vi "FGV ARN Daten.vi"(0 "ARN Konfig Daten":T1={"Bearbeiter:"="", "Analysator"="FT-IR", "Komponente:"=0, "Gasflaschen Nr.:"="", "Accuracy"=0.0, "Sollwert"=0.0, "Modus"=0, "Pfad:"=path "D:/IAG_Data/Log", "Textname:"="", "CG Aufschaltzeit:"=120.0, "Einheit"="", "N2 Aufschaltzeit:"=120.0, "Gasflasche"=0, "Konfig Gasflasche"=FALSE} {"Gasflasche" items=["----"=10000, "IAG NH3 3000"=0, "IAG NH3 200"=1, "IAG NH3 2000"=2, "IAG MG"=3, "IAG O2"=4]; "Komponente:" items=["NO (350,3000) LP 191C", "NO2 (150) LP 191C (1of2)", "NO2 (2000) LP 191C (2of2)", "N2O (300) LP 191C (1of2)", "NH3 (300) LP 191C (1of2)", "NH3 (900,3000) LP 191C (2of2)", "HNCO (400) 191C", "H2O% (30) LP 191C", "Formaldehyde (70,500) LP 191C", "CO2 low% (4) LP 191C (2of2)", "CO2% (20) LP 191C (1of2)", "CO (700) LP 191C (1of3)", "CO% (1) LP 191C (2of3)", "Propylene (1000) LP 191C", "Aromatic HC C7 (500) LP 191C", "Ethylene (1000) LP 191C", "CH4 (250) LP 191C (1of2)", "CH4 (5000) LP 191C (2of2)", "Ethane (1000) LP 191C", "Acetylene (1000) LP 191C", "HNO2 (20) 191C", "MeOH (1000) 191C", "CO% (10) LP 191C (3of3)", "Formic Acid (100) 191C", "SO2 (500) LP 191C", "Acetaldehyde (1000) LP 191C", "COS (100) LP 191C", "1,3 butadiene (100) LP 191C", "Oil as Octane (200) LP 191C", "N2O (1000) LP 191C (2of2)", "Propane (200) LP 191C", "NO2 autorange (2000)", "CO autorange (100000)", "CH4 autorange (5000)", "NH3 autorange (3000)", "Temp. Gascell", "Pressure Gascell", "sBeam@2500"]; "Modus" items=["CG zu PNS", "CG zu Entnahmestelle"]; "N2 Aufschaltzeit:" min=10.0; "CG Aufschaltzeit:" min=10.0}, 1 "N2":bool, 5 "Rohdaten":sgl[](array[numeric]), 7 "Zeitstempel":string, 9 "SNR Ergebnis":sgl[](array[numeric]), 11 "error in (no error)":errorcluster caption="Fehler (Eingang, kein Fehler)", 12 "Aktion":T6) -> (4 "ARN Konfig Daten":T1={"Bearbeiter:"="", "Analysator"="FT-IR", "Komponente:"=0, "Gasflaschen Nr.:"="", "Accuracy"=0.0, "Sollwert"=0.0, "Modus"=0, "Pfad:"=path "D:/IAG_Data/Log", "Textname:"="", "CG Aufschaltzeit:"=120.0, "Einheit"="", "N2 Aufschaltzeit:"=120.0, "Gasflasche"=0, "Konfig Gasflasche"=FALSE} {"Gasflasche" items=["----"=10000, "IAG NH3 3000"=0, "IAG NH3 200"=1, "IAG NH3 2000"=2, "IAG MG"=3, "IAG O2"=4]; "Komponente:" items=["NO (350,3000) LP 191C", "NO2 (150) LP 191C (1of2)", "NO2 (2000) LP 191C (2of2)", "N2O (300) LP 191C (1of2)", "NH3 (300) LP 191C (1of2)", "NH3 (900,3000) LP 191C (2of2)", "HNCO (400) 191C", "H2O% (30) LP 191C", "Formaldehyde (70,500) LP 191C", "CO2 low% (4) LP 191C (2of2)", "CO2% (20) LP 191C (1of2)", "CO (700) LP 191C (1of3)", "CO% (1) LP 191C (2of3)", "Propylene (1000) LP 191C", "Aromatic HC C7 (500) LP 191C", "Ethylene (1000) LP 191C", "CH4 (250) LP 191C (1of2)", "CH4 (5000) LP 191C (2of2)", "Ethane (1000) LP 191C", "Acetylene (1000) LP 191C", "HNO2 (20) 191C", "MeOH (1000) 191C", "CO% (10) LP 191C (3of3)", "Formic Acid (100) 191C", "SO2 (500) LP 191C", "Acetaldehyde (1000) LP 191C", "COS (100) LP 191C", "1,3 butadiene (100) LP 191C", "Oil as Octane (200) LP 191C", "N2O (1000) LP 191C (2of2)", "Propane (200) LP 191C", "NO2 autorange (2000)", "CO autorange (100000)", "CH4 autorange (5000)", "NH3 autorange (3000)", "Temp. Gascell", "Pressure Gascell", "sBeam@2500"]; "Modus" items=["CG zu PNS", "CG zu Entnahmestelle"]; "N2 Aufschaltzeit:" min=10.0; "CG Aufschaltzeit:" min=10.0}, 6 "Rohdaten":sgl[][](array[numeric]), 8 "Zeitstempel":string, 10 "SNR Ergebnis":sgl[](array[numeric]), 14 "Rohdaten N2":sgl[][](array[numeric]), 15 "error out":errorcluster caption="Fehler (Ausgang)")   [LabVIEW 2020, in "EPA 1065.lvlib" / "ARN Test 1065-305.lvlib"]
uses:
  ARN Test 1065-305.lvlib
  Aktion FGV ARN Daten.ctl
  Allgemeine Einstellungen.ctl
  Seiten/System Einstellungen V2/Analysatoren.ctl
  T90 1065-308/Modus.ctl
  Seiten/System Einstellungen V2/Gasflasche Auswahl.ctl
  Seiten/System Einstellungen V2/Konfig Gasflasche.ctl
  Allgemein/allgemeine Sub-VIs.lvlib
  T90 1065-308/T90 Test 1065-308.lvlib
  Seiten/System Einstellungen V2/System Einstellungen V2.lvlib
panel:
  # "%"
  # "sec."
  # "sec."
  # "%"
  # "sec."
  # "sec."
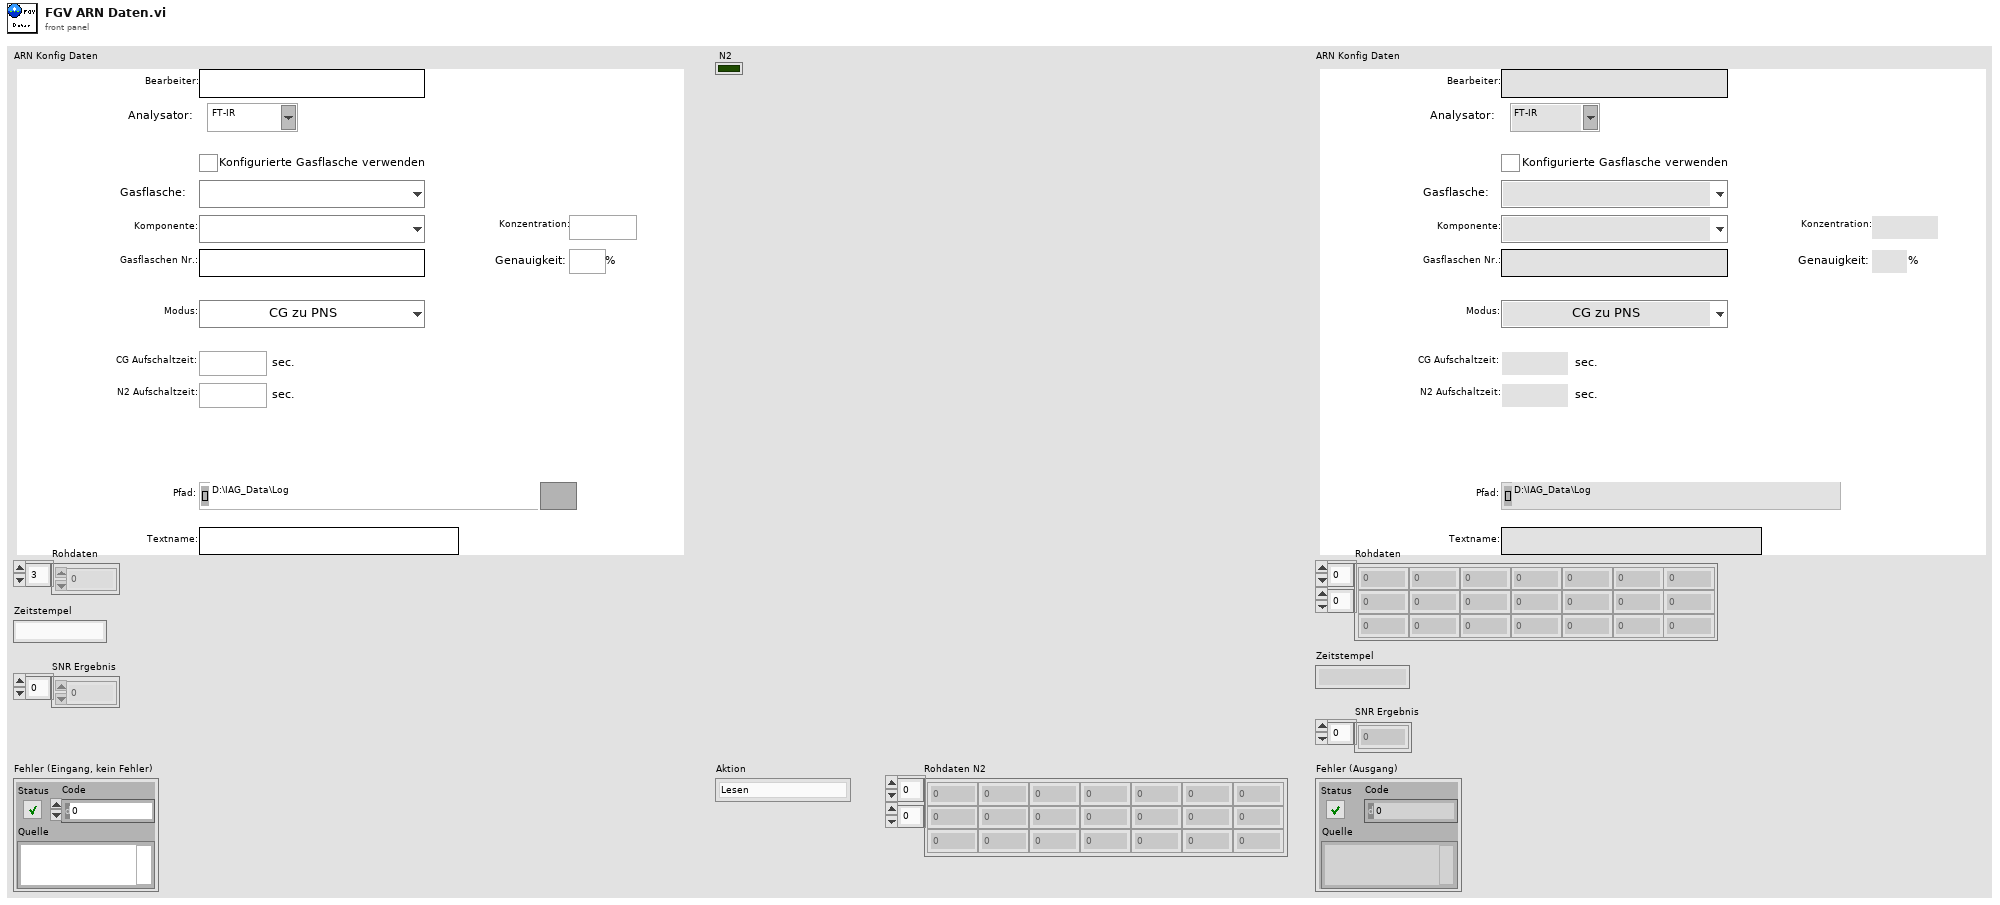
[diagram p1: front panel]
types:
  T1 = typedef "EPA 1065.lvlib/ARN Test 1065-305.lvlib/Allgemeine Einstellungen.ctl" = cluster{"Bearbeiter:":string, "Analysator":T2, "Komponente:":u16, "Gasflaschen Nr.:":string, "Accuracy":dbl, "Sollwert":dbl, "Modus":T3, "Pfad:":path, "Textname:":string, "CG Aufschaltzeit:":dbl, "Einheit":string, "N2 Aufschaltzeit:":dbl, "Gasflasche":T4, "Konfig Gasflasche":T5}
  T2 = typedef "System Einstellungen V2.lvlib/Analysatoren.ctl" = string
  T3 = typedef "EPA 1065.lvlib/T90 Test 1065-308.lvlib/Modus.ctl" = u16
  T4 = typedef "System Einstellungen V2.lvlib/Gasflasche Auswahl.ctl" = u16
  T5 = typedef "System Einstellungen V2.lvlib/Konfig Gasflasche.ctl" = bool
  T6 = typedef "EPA 1065.lvlib/ARN Test 1065-305.lvlib/Aktion FGV ARN Daten.ctl" = enum16{"Lesen", "laden", "speichern", "ARN Daten", "Rohdaten", "Rohdaten löschen", "Zeitstempel", "SNR Ergebnis"}
  T7 = enum16{"open", "replace", "create", "open or create", "replace or create", "replace or create with confirmation"}
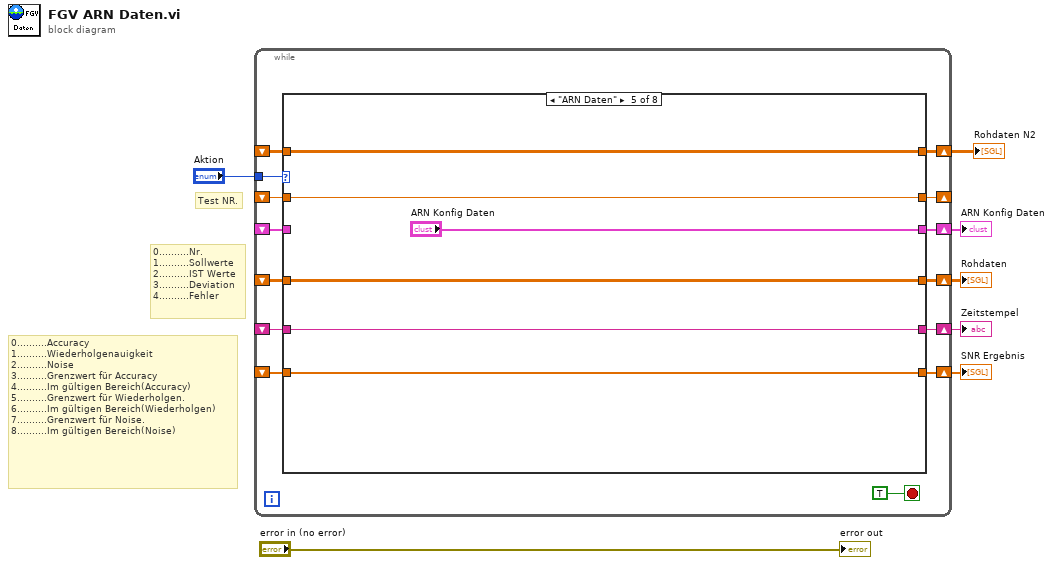
[diagram p0: block diagram]
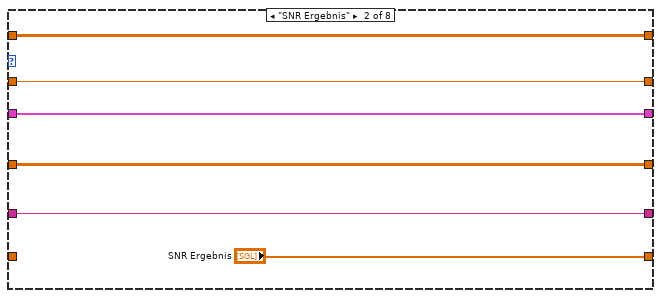
[diagram p3: hidden frame]
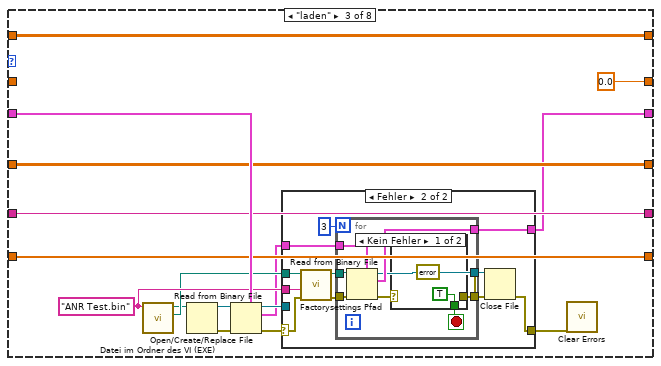
[diagram p4: hidden frame]
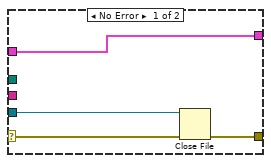
[diagram p5: hidden frame]
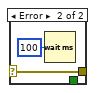
[diagram p6: hidden frame]
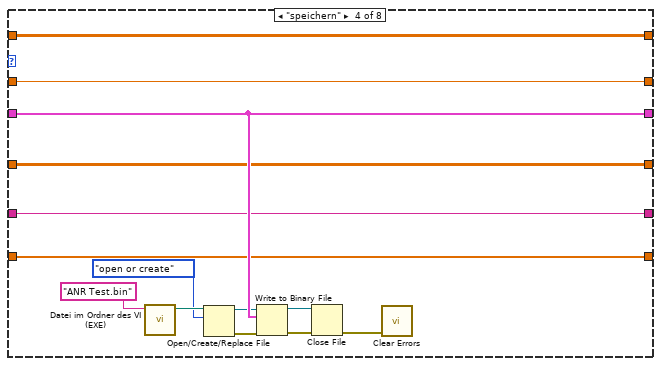
[diagram p7: hidden frame]
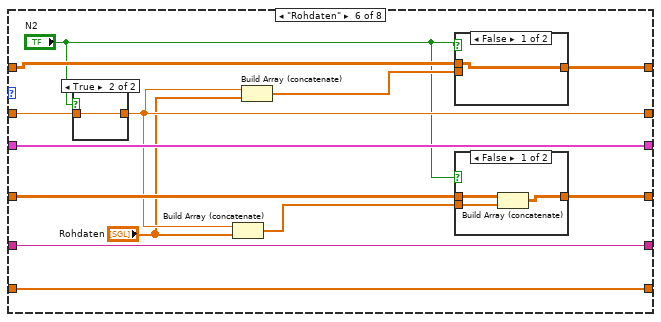
[diagram p8: hidden frame]
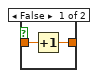
[diagram p10: hidden frame]
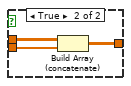
[diagram p11: hidden frame]
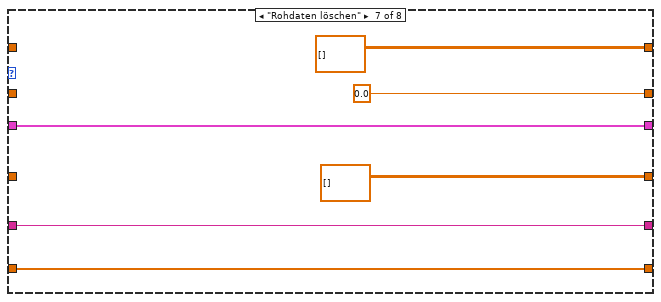
[diagram p12: hidden frame]
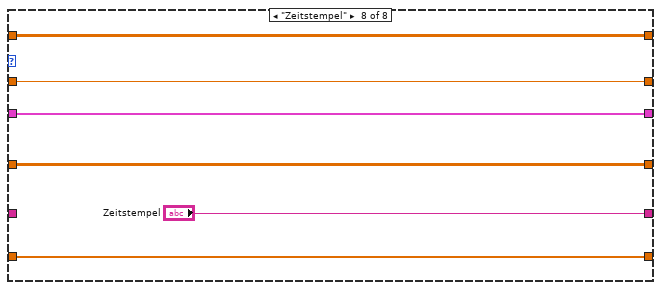
[diagram p13: hidden frame]
diagram:
  # "Test NR."
  # "0..........Accuracy\n1..........Wiederholgenauigkeit\n2..........Noise\n3..........Grenzwert für Accuracy\n4..........Im gültigen Bereich(Accuracy)\n5..........Grenzwert für Wiederholgen.\n6..........Im gültigen Bereich(Wiederholgen)\n7..........Grenzwert für Noise.\n8..........Im gültigen Bereich(Noise)"
  # "0..........Nr.\n1..........Sollwerte\n2..........IST Werte\n3..........Deviation\n4..........Fehler"
  n1 = while {
    tunnel: "Aktion" -> [w20]
    shift-right: [w19] -> w6
    shift-left: _ -> [w18]
    shift-right: [w17] -> w5
    shift-left: _ -> [w16]
    shift-right: [w15] -> w4
    shift-left: _ -> [w14]
    shift-right: [w13] -> w3
    shift-left: _ -> [w12]
    shift-right: [w11] -> _
    shift-left: _ -> [w10]
    shift-right: [w9] -> w1
    shift-left: _ -> [w8]
    stop <- TRUE stop-if-true
    n2 = case shown="\"ARN Daten\"" w20 {
      tunnel: [w27 w33 w38 w89 "ARN Konfig Daten" w109 w126 w132] -> w19
      tunnel: w18 -> [w27 w33 w49 w89 _ w109 w126 w132]
      tunnel: [w26 w32 w48 w88 w95 w103 sgl[][] [] ("Rohdaten") w131] -> w17
      tunnel: w16 -> [w26 w32 w48 w88 w95 w108 _ w131]
      tunnel: [w25 w31 w47 w87 w94 w107 w124 "Zeitstempel"] -> w15
      tunnel: w14 -> [w25 w31 w47 w87 w94 w107 w124 _]
      tunnel: [w24 "SNR Ergebnis" w46 w86 w93 w106 w123 w129] -> w13
      tunnel: w12 -> [w24 _ w46 w86 w93 w106 w123 w129]
      tunnel: [w23 w29 sgl 0.0 w85 w92 w102 sgl 0.0 w128] -> w11
      tunnel: w10 -> [w23 w29 _ w85 w92 w104 _ w128]
      tunnel: [w22 w28 w37 w84 w91 w99 sgl[][] [] w127] -> w9
      tunnel: w8 -> [w22 w28 w37 w84 w91 w98 _ w127]
      frame "Lesen", Default {
      }
      frame "SNR Ergebnis" {
      }
      frame "laden" {
        w42 = "ANR Test.bin" ("Dateiname")
        n3 = call "Datei im Ordner des VI (EXE).vi"("Dateiname"=w42) -> ("Ordner des Haupt-VIs"=w41:path, "Dateipfad im Ordner des Haupt-VIs"=w36:path)  [unwired: 8 in, 1 out]
        n4 = Open/Create/Replace File(file path (use dialog)=w36) -> (refnum out=w34:refnum<file>, error out=w35:errorcluster)  [unwired: 5 in, 1 out]
        n5 = Read from Binary File(5:w49, 8:w35, 11:w34) -> (0:w44:errorcluster, 2:w39:T1, 3:w40:refnum<file>)  [unwired: 3 in, 1 out]
        n6 = case shown="Fehler" w44 {
          selector: w44 -> [w52 w56]
          tunnel: w41 -> [_ w57]
          tunnel: w39 -> [w53 w55]
          tunnel: [w53 w63] -> w38
          tunnel: [w50 w61] -> w43
          tunnel: w40 -> [w51 _]
          tunnel: w42 -> [_ w54]
          frame No Error {
            n7 = Close File(refnum=w51, error in=w52) -> (error out=w50:errorcluster)  [unwired: 1 out]
          }
          frame Error {
            n8 = call "Factorysettings Pfad.vi"("error in (no error)"=w56, "Dateiname"=w54, "Ordner des Haupt-VIs"=w57) -> ("error out"=w58:errorcluster, "Pfad Factorysettings"=w59:path)  [unwired: 7 in]
            n9 = for {
              N: 3 -> [_]
              tunnel: w58 -> [w70]
              tunnel: w59 -> [w69]
              tunnel: [w68] -> w63
              tunnel: [w67] -> w62
              tunnel: [w66] -> w60
              tunnel: w55 -> [w65]
              stop <- w71 stop-if-true
              n10 = Read from Binary File(5:w65, 8:w70, 11:w69) -> (0:w72:errorcluster, 2:w68:T1, 3:w66:refnum<file>)  [unwired: 3 in, 1 out]
              n11 = case shown="Kein Fehler" w72 {
                selector: w72 -> [_ w75]
                tunnel: [TRUE _] -> w71
                tunnel: [errorcluster {"status"=FALSE, "code"=0, "source"=""} ("error IO") w75] -> w67
                frame No Error {
                }
                frame Error {
                  n12 = Wait (ms)(milliseconds to wait=u32 100 ("Zu wartende ms")) -> ()  [unwired: 1 out]
                }
              }
            }
            n13 = Close File(refnum=w60, error in=w62) -> (error out=w61:errorcluster)  [unwired: 1 out]
          }
        }
        n14 = call <vilib>:"Clear Errors.vi"("error in (no error)"=w43) -> ()  [unwired: 5 in, 2 out]
      }
      frame "speichern" {
        n15 = call "Datei im Ordner des VI (EXE).vi"("Dateiname"="ANR Test.bin") -> ("Dateipfad im Ordner des Haupt-VIs"=w82:path)  [unwired: 8 in, 2 out]
        n16 = Open/Create/Replace File(file path (use dialog)=w82, operation (0:open)=T7."open or create" ("Operation (0:Öffnen)")) -> (refnum out=w81:refnum<file>, error out=w83:errorcluster)  [unwired: 4 in, 1 out]
        n17 = Write to Binary File(file (use dialog)=w81, data=w89, error in=w83) -> (refnum out=w80:refnum<file>, error out=w79:errorcluster)  [unwired: 3 in, 1 out]
        n18 = Close File(refnum=w80, error in=w79) -> (error out=w78:errorcluster)  [unwired: 1 out]
        n19 = call <vilib>:"Clear Errors.vi"("error in (no error)"=w78) -> ()  [unwired: 5 in, 2 out]
      }
      frame "ARN Daten" {
      }
      frame "Rohdaten" {
        n20 = case shown="True" "N2" {
          tunnel: w104 -> [w115 w116]
          tunnel: [w114 w116] -> w102
          frame False {
            n21 = Increment(x=w115) -> (x+1=w114:sgl)
          }
          frame True {
          }
        }
        n22 = Build Array (concatenate)(w102, "Rohdaten") -> (w105:sgl[])
        n23 = Build Array (concatenate)(w102, "Rohdaten") -> (w100:sgl[])
        n24 = case shown="False" "N2" {
          tunnel: w100 -> [_ w120]
          tunnel: [w117 w119] -> w99
          tunnel: w98 -> [w117 w118]
          frame False {
          }
          frame True {
            n25 = Build Array (concatenate)(w118, w120) -> (w119:sgl[][])
          }
        }
        n26 = case shown="False" "N2" {
          tunnel: w108 -> [w112 w113]
          tunnel: w105 -> [w111 _]
          tunnel: [w110 w113] -> w103
          frame False {
            n27 = Build Array (concatenate)(w112, w111) -> (w110:sgl[][])
          }
          frame True {
          }
        }
      }
      frame "Rohdaten löschen" {
      }
      frame "Zeitstempel" {
      }
    }
  }
  "ARN Konfig Daten" <- w6
  "Rohdaten" <- w5
  "Zeitstempel" <- w4
  "SNR Ergebnis" <- w3
  "Rohdaten N2" <- w1
  "error out" <- "error in (no error)"
